vi "Field Add.vi"(8 "error in (no error)":errorcluster, 9 "Force Unique? (f)":bool, 10 "Field Record":T1={"ixField"=0, "iSequenceOrder"=0, "sxFieldId"="", "sxSequenceId"="", "sDisplayName"="", "sValue"="", "sUnits"="", "nDataType"=enum."timestamp", "nNextItem"=enum."Reset", "fSystem"=FALSE, "fSystemValue"=FALSE, "fRequired"=FALSE, "fSetAtTest"=FALSE, "fTestField"=FALSE, "fDeleted"=FALSE, "fIndexed"=FALSE, "fFreeList"=FALSE}, 11 "Connection Refnum":T4) -> (0 "error out":errorcluster, 2 "New Field":T1={"ixField"=0, "iSequenceOrder"=0, "sxFieldId"="", "sxSequenceId"="", "sDisplayName"="", "sValue"="", "sUnits"="", "nDataType"=enum."timestamp", "nNextItem"=enum."Reset", "fSystem"=FALSE, "fSystemValue"=FALSE, "fRequired"=FALSE, "fSetAtTest"=FALSE, "fTestField"=FALSE, "fDeleted"=FALSE, "fIndexed"=FALSE, "fFreeList"=FALSE}, 3 "Connection Refnum":T4)   [LabVIEW 2011]
uses:
  Field Record.ctl
  Field DataTypes.ctl
  Field NextItem.ctl
  SI.LIB/ODBC/SQL Controls/Connection Refnum.ctl
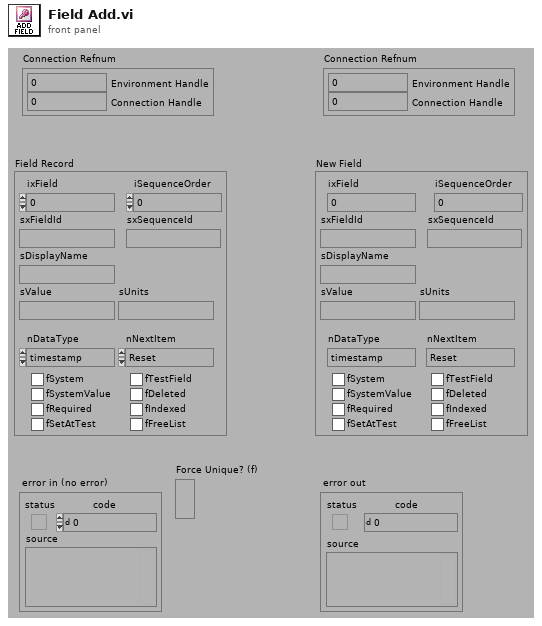
[diagram p1: front panel]
types:
  T1 = typedef "Field Record.ctl" = cluster{"ixField":i32, "iSequenceOrder":i32, "sxFieldId":string, "sxSequenceId":string, "sDisplayName":string, "sValue":string, "sUnits":string, "nDataType":T2, "nNextItem":T3, "fSystem":bool, "fSystemValue":bool, "fRequired":bool, "fSetAtTest":bool, "fTestField":bool, "fDeleted":bool, "fIndexed":bool, "fFreeList":bool}
  T2 = typedef "Field DataTypes.ctl" = enum32{"text", "numeric", "list", "timestamp", "boolean"}
  T3 = typedef "Field NextItem.ctl" = enum32{"Reset", "Retain", "Auto-Increment"}
  T4 = typedef "Connection Refnum.ctl" = cluster{"Environment Handle":i32, "Connection Handle":i32}
  T5 = typedef "Statement Refnum.ctl" = cluster{"Statement Handle":i32, "Parameter Number":u16}
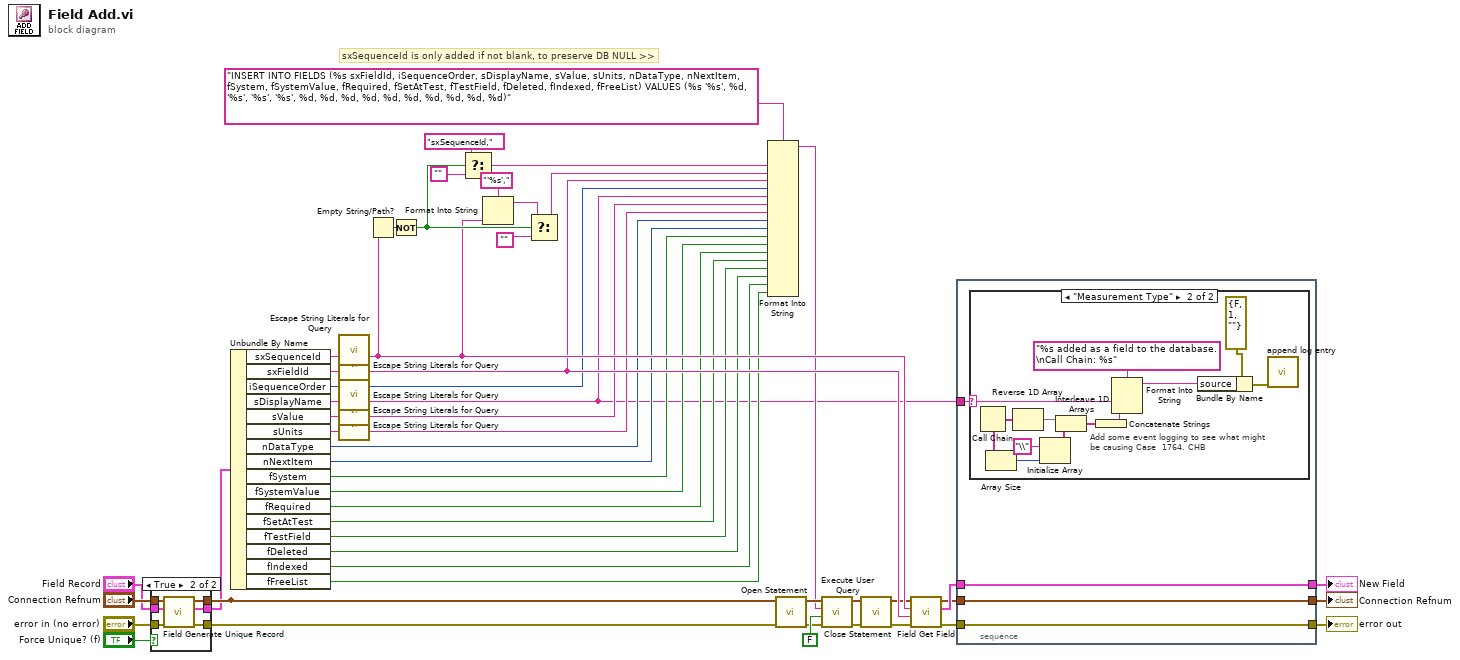
[diagram p0: block diagram]
diagram:
  # "sxSequenceId is only added if not blank, to preserve DB NULL >>"
  n1 = case shown="True" "Force Unique? (f)" {
    tunnel: "Connection Refnum" -> [w54 w59]
    tunnel: "error in (no error)" -> [w53 w58]
    tunnel: [w54 w57] -> w15
    tunnel: [w53 w56] -> w14
    tunnel: "Field Record" -> [w52 w60]
    tunnel: [w52 w55] -> w10
    frame False {
    }
    frame True {
      n2 = call "Field Generate Unique Record.vi"("error in (no error)"=w58, "Field Record (empty)"=w60, "Connection Refnum"=w59) -> ("error out"=w56:errorcluster, "Unique Field Record"=w55:T1, "Connection Refnum"=w57:T4)  [unwired: 6 out]
    }
  }
  n3 = Unbundle By Name(w10) -> ("sxSequenceId"=w44:string, "sxFieldId"=w13:string, "iSequenceOrder"=w32:i32, "sDisplayName"=w12:string, "sValue"=w31:string, "sUnits"=w29:string, "nDataType"=w27:T2, "nNextItem"=w26:T3, "fSystem"=w25:bool, "fSystemValue"=w24:bool, "fRequired"=w23:bool, "fSetAtTest"=w22:bool, "fTestField"=w21:bool, "fDeleted"=w20:bool, "fIndexed"=w9:bool, "fFreeList"=w8:bool)
  n4 = call "Escape String Literals for Query.vi"("String"=w44) -> ("escaped String"=w35:string)  [unwired: 1 in, 13 out]
  n5 = call "Escape String Literals for Query.vi"("String"=w13) -> ("escaped String"=w33:string)  [unwired: 1 in, 13 out]
  n6 = call "Escape String Literals for Query.vi"("String"=w12) -> ("escaped String"=w7:string)  [unwired: 1 in, 13 out]
  n7 = call "Escape String Literals for Query.vi"("String"=w31) -> ("escaped String"=w30:string)  [unwired: 1 in, 13 out]
  n8 = call "Escape String Literals for Query.vi"("String"=w29) -> ("escaped String"=w28:string)  [unwired: 1 in, 13 out]
  n9 = Empty String/Path?(string/path=w35) -> (empty?=w46:bool)
  n10 = Not(x=w46) -> (.not. x?=w38:bool)
  n11 = Select(t="sxSequenceId," ("User Query"), s=w38, f="") -> (s? t:f=w36:string)
  n12 = Format Into String(format string="'%s'," ("User Query"), w35) -> (resulting string=w41:string)  [unwired: 2 in, 1 out]
  n13 = Select(t=w41, s=w38, f="") -> (s? t:f=w34:string)
  n14 = Format Into String(format string="INSERT INTO FIELDS (%s sxFieldId, iSequenceOrder, sDisplayName, sValue, sUnits, nDataType, nNextItem, fSystem, fSystemValue, fRequired, fSetAtTest, fTestField, fDeleted, fIndexed, fFreeList) VALUES (%s '%s', %d, '%s', '%s', '%s', %d, %d, %d, %d, %d, %d, %d, %d, %d, %d)" ("User Query"), w36, w34, w33, w32, w7, w30, w28, w27, w26, w25, w24, w23, w22, w21, w20, w9, w8) -> (resulting string=w19:string)  [unwired: 2 in, 1 out]
  n15 = call "Open Statement.vi"("error in (no error)"=w14, "Connection Refnum"=w15) -> ("error out"=w48:errorcluster, "Statement Refnum"=w47:T5)  [unwired: 4 out]
  n16 = call "Execute User Query.vi"("error in (no error)"=w48, "Return Data? (f)"=FALSE, "User Query"=w19, "Statement Refnum"=w47) -> ("error out"=w49:errorcluster, "Statement Refnum"=w50:T5)  [unwired: 2 out]
  n17 = call "Close Statement.vi"("error in (no error)"=w49, "Statement Refnum"=w50) -> ("error out"=w45:errorcluster)  [unwired: 5 out]
  n18 = call "Field Get Field.vi"("error in (no error)"=w45, "sFieldId or sDisplayName (\"\")"=w33, "sxSequenceId (\"\")"=w35, "Connection Refnum"=w15) -> ("error out"=w4:errorcluster, "Field"=w6:T1, "Connection Refnum"=w5:T4)  [unwired: 1 in, 4 out]
  n19 = stacked-sequence {
    tunnel: w7 -> [w61]
    tunnel: w6 -> [w64]
    tunnel: w5 -> [w63]
    tunnel: w4 -> [w62]
    tunnel: [w64] -> w3
    tunnel: [w63] -> w2
    tunnel: [w62] -> w1
    frame #0 {
      n20 = case shown="\"Measurement Type\"" w61 {
        selector: w61 -> [_ w72]
        frame Default {
        }
        frame "Measurement Type" {
          # "Add some event logging to see what might\nbe causing Case  1764. CHB"
          n21 = Call Chain() -> (call chain=w69:string[])
          n22 = Array Size(array=w69) -> (size(s)=w71:i32)
          n23 = Reverse 1D Array(array=w69) -> (reversed array=w68:string[])
          n24 = Initialize Array("\\" ("format string"), w71) -> (w67:string[])
          n25 = Interleave 1D Arrays(w68, w67) -> (w66:string[])
          n26 = Concatenate Strings(w66) -> (w65:string)
          n27 = Format Into String(format string="%s added as a field to the database.\nCall Chain: %s", w72, w65) -> (resulting string=w74:string)  [unwired: 2 in, 1 out]
          n28 = Bundle By Name(cluster=errorcluster {"status"=FALSE, "code"=1, "source"=""} ("error in (no error)"), "source"=w74) -> (w73:errorcluster)
          n29 = call "append log entry.vi"("error in (no error)"=w73) -> ()  [unwired: 9 in, 1 out]
        }
      }
    }
  }
  "error out" <- w1
  "Connection Refnum" <- w2
  "New Field" <- w3
